vi "Arm3D.vi"() -> ()   [LabVIEW 2024]
uses:
  <vilib>/Native 3D Graph/xcontrol/3DPC_SurfacePlot.xctl
  <vilib>/Utility/miscctls.llb/LV3DPointTypeDef.ctl
  <vilib>/Analysis/Matrix/Datatypes/RealMatrix.ctl
  <vilib>/Analysis/baseanly.llb/Real A x B.vi
  <vilib>/Analysis/NI_AALBase.lvlib
  <vilib>/Analysis/Matrix/NI_Matrix.lvlib
panel:
  out "2D Picture":picture
  out "3D Graph":refnum<class "Base Datatype.lvclass">[](xcontrol)
  out "3D Picture":refnum<vi>(3d-picture)
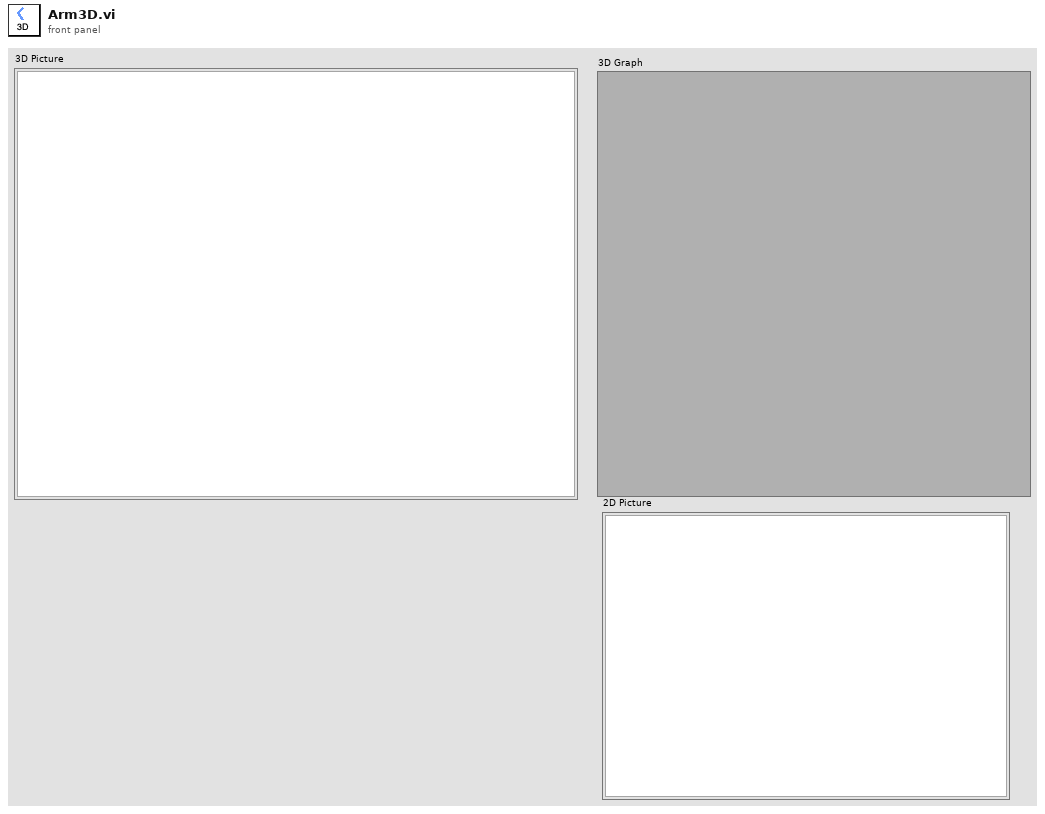
[diagram p1: front panel]
types:
  T1 = typedef "NI_Matrix.lvlib/RealMatrix.ctl" = dbl[][]
  T2 = typedef "LV3DPointTypeDef.ctl" = cluster{"X":sgl, "Y":sgl, "Z":sgl}
  T3 = enum16{"None", "Spherical", "Flying", "Oriented"}
  T4 = cluster{"Line width":sgl, "Line Color":u32, "Axes?":bool}
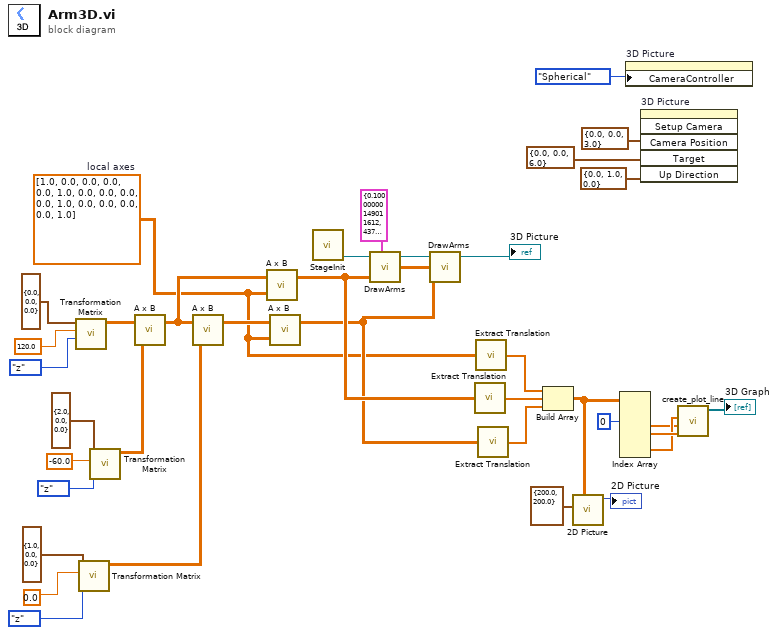
[diagram p0: block diagram]
diagram:
  w1 = T1 [[1.0, 0.0, 0.0, 0.0], [0.0, 1.0, 0.0, 0.0], [0.0, 0.0, 1.0, 0.0], [0.0, 0.0, 0.0, 1.0]]  # local axes
  n1 = call <userlib>:"Transformation Matrix.vi"("Axis"=enum16{"x", "y", "z"}."z", "Angle (degrees)"=120.0, "Translation"=cluster{"X":dbl, "Y":dbl, "Z":dbl} {"X"=0.0, "Y"=0.0, "Z"=0.0}) -> ("Transformation Matrix"=w10:T1)  [unwired: 8 in]
  n2 = call <userlib>:"Transformation Matrix.vi"("Axis"=enum16{"x", "y", "z"}."z", "Angle (degrees)"=0.0, "Translation"=cluster{"X":dbl, "Y":dbl, "Z":dbl} {"X"=1.0, "Y"=0.0, "Z"=0.0}) -> ("Transformation Matrix"=w19:T1)  [unwired: 8 in]
  n3 = call <userlib>:"Transformation Matrix.vi"("Axis"=enum16{"x", "y", "z"}."z", "Angle (degrees)"=-60.0, "Translation"=cluster{"X":dbl, "Y":dbl, "Z":dbl} {"X"=2.0, "Y"=0.0, "Z"=0.0}) -> ("Transformation Matrix"=w20:T1)  [unwired: 8 in]
  n4 = call-poly <vilib>:"A x B.vi"("B"=w20, "A"=w10) -> ("A x B"=w5:T1)  [unwired: 1 out]
  n5 = call-poly <vilib>:"A x B.vi"("B"=w19, "A"=w5) -> ("A x B"=w3:T1)  [unwired: 1 out]
  n6 = call-poly <vilib>:"A x B.vi"("B"=w1, "A"=w5) -> ("A x B"=w4:T1)  [unwired: 1 out]
  n7 = call-poly <vilib>:"A x B.vi"("B"=w1, "A"=w3) -> ("A x B"=w2:T1)  [unwired: 1 out]
  n8 = call <userlib>:"StageInit.vi"() -> ("Stage out"=w34:refnum<vi>)  [unwired: 4 in, 1 out]
  n9 = call <userlib>:"DrawArms.vi"("Stage in"=w34, "Params"=T4 {"Line width"=0.1, "Line Color"=4376575, "Axes?"=TRUE}, "End"=w4) -> ("Stage out"=w9:refnum<vi>, "End Out"=w7:T1)  [unwired: 3 in]
  n10 = call <userlib>:"DrawArms.vi"("Stage in"=w9, "Start"=w7, "End"=w2) -> ("Stage out"=→"3D Picture":refnum<vi>)  [unwired: 3 in, 1 out]
  n11 = call <userlib>:"Extract Translation.vi"("Transformation matrix"=w4) -> ("translation"=w17:dbl[])
  n12 = call <userlib>:"Extract Translation.vi"("Transformation matrix"=w1) -> ("translation"=w30:dbl[])
  n13 = call <userlib>:"Extract Translation.vi"("Transformation matrix"=w2) -> ("translation"=w16:dbl[])
  n14 = Build Array(w30, w17, w16) -> (w11:dbl[][])
  n15 = call <userlib>:"2D Picture.vi"("position array"=w11, "Origin"=cluster{"x":dbl, "y":dbl} {"x"=200.0, "y"=200.0}) -> ("picture out"=→"2D Picture":picture)  [unwired: 9 in]
  n16 = Index Array(array=w11, index (col) #1=0 ("disabled index (col)")) -> (element #1=w27:dbl[], element #2=w29:dbl[], element #3=w28:dbl[])  [unwired: 5 in]
  n17 = property on="3D Picture" class="SceneGraphDisp (strict)"("CameraController"=T3."Spherical" ("Camera Controller:Type")) -> ()  [unwired: 2 in, 2 out]
  n18 = invoke on="3D Picture" class="SceneGraphDisp (strict)" method="Setup Camera"("Camera Position"=T2 {"X"=0.0, "Y"=0.0, "Z"=6.0}, "Target"=T2 {"X"=0.0, "Y"=0.0, "Z"=3.0}, "Up Direction"=T2 {"X"=0.0, "Y"=1.0, "Z"=0.0}) -> ()  [unwired: 3 in, 6 out]
  n19 = call <vilib>:"create_plot_line.vi"("z vector"=w29, "y vector"=w27, "x vector"=w28) -> ("plots out"=→"3D Graph":refnum<class "Base Datatype.lvclass">[])  [unwired: 2 in, 6 out]
